vi "reentrantRationalResample.vi"(0 "X":sgl[][](array[numeric]), 1 "reset":bool, 7 "resample factor":cluster{"interpolation":i32, "decimation":i32}, 11 "error in (no error)":errorcluster) -> (4 "Y":dbl[][](array[numeric]), 15 "error out":errorcluster)   [LabVIEW 2017, in "BufferLogging.lvlib"]
uses:
  BufferLogging.lvlib
  <vilib>/Analysis/2dsp.llb/Rational Resample (multi-channel, DBL).vi
  <vilib>/Analysis/NI_AALPro.lvlib
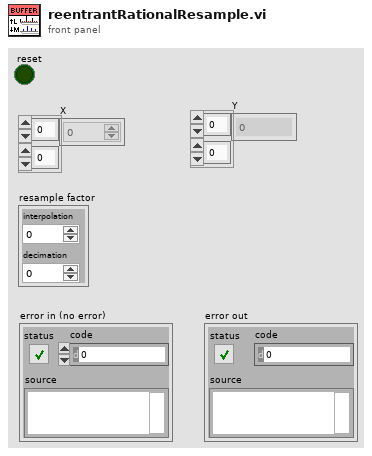
[diagram p1: front panel]
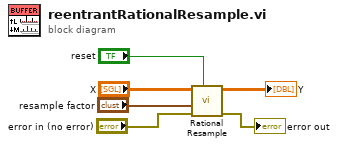
[diagram p0: block diagram]
diagram:
  n1 = call-poly <vilib>:"Rational Resample.vi"("reset"="reset", "error in (no error)"="error in (no error)", "resample factor"="resample factor", "X"="X") -> ("error out"=→"error out":errorcluster, "Y"=→"Y":dbl[][])  [unwired: 5 in, 1 out]
